vi "Build Description String.vi"(8 "error in (no error)":errorcluster, 11 "Macro Step in":refnum<class "Macro Step.lvclass">) -> (0 "error out":errorcluster, 2 "Description":string, 3 "Macro Step out":refnum<class "Macro Step.lvclass">)   [LabVIEW 2020, in "MacroAssert.lvlib" / "Macro Step.lvclass"]
doc: "Builds a string to describe what <B>Step</B> does."
uses:
  Macro Step.lvclass
  Macro Step.lvclass/Macro Step.ctl
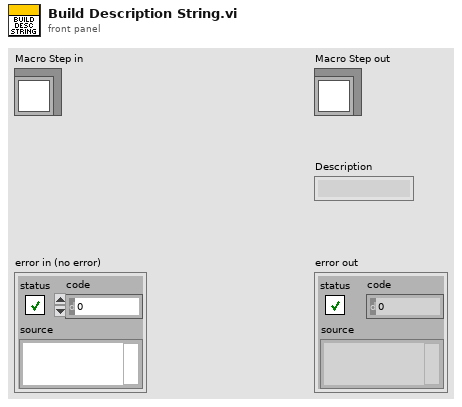
[diagram p1: front panel]
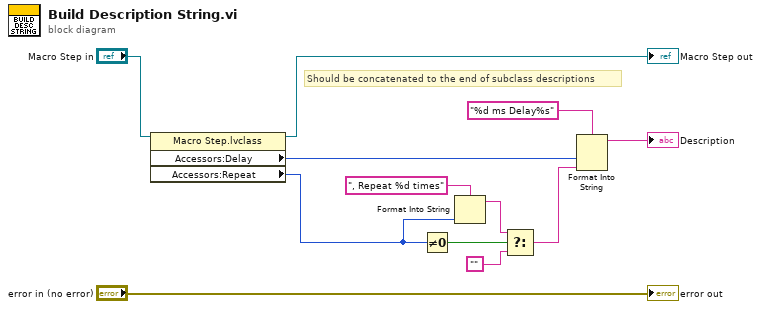
[diagram p0: block diagram]
diagram:
  # "Should be concatenated to the end of subclass descriptions"
  n1 = property class="Macro Step.lvclass"(reference="Macro Step in") -> (reference out=→"Macro Step out":refnum<class "Macro Step.lvclass">, "Accessors:Delay"=w3:i32, "Accessors:Repeat"=w4:i32)  [unwired: 1 in, 1 out]
  n2 = Not Equal To 0?(x=w4) -> (x != 0?=w11:bool)
  n3 = Format Into String(format string=", Repeat %d times", w4) -> (resulting string=w10:string)  [unwired: 2 in, 1 out]
  n4 = Select(t=w10, s=w11, f="") -> (s? t:f=w2:string)
  n5 = Format Into String(format string="%d ms Delay%s", w3, w2) -> (resulting string=→"Description":string)  [unwired: 2 in, 1 out]
  "error out" <- "error in (no error)"
